vi "HouseBlend.vi"(8 "error in (no error)":errorcluster caption="错误输入（无错误）", 11 "House Blend Coffee 输入":refnum<class "House Blend Coffee.lvclass">) -> (0 "error out":errorcluster caption="错误输出", 3 "House Blend Coffee 输出":refnum<class "House Blend Coffee.lvclass">)   [LabVIEW 2016, in "House Blend Coffee.lvclass"]
uses:
  House Blend Coffee.lvclass
  Beverage.lvclass/Beverage.ctl
  Beverage.lvclass
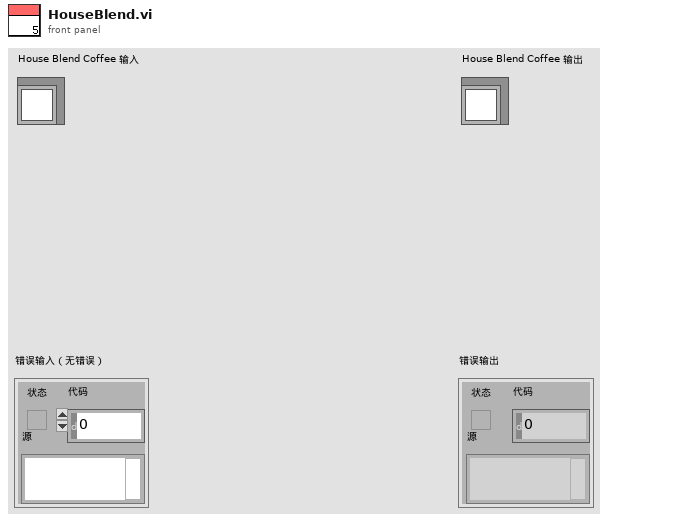
[diagram p1: front panel]
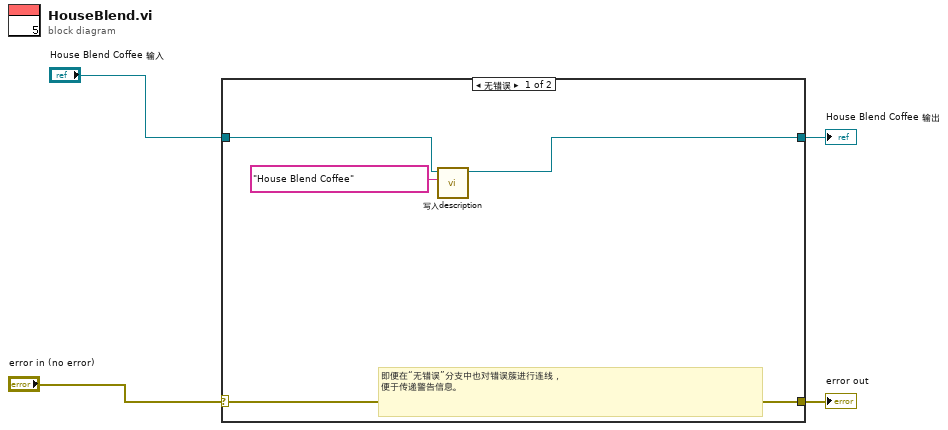
[diagram p0: block diagram]
diagram:
  n1 = case shown="无错误" "error in (no error)" {
    selector: "error in (no error)" -> [w8 w10]
    tunnel: [w8 w10] -> w3
    tunnel: [w6 w9] -> w1
    tunnel: "House Blend Coffee 输入" -> [w7 w9]
    frame No Error {
      # "即便在“无错误”分支中也对错误簇进行连线，\n便于传递警告信息。"
      n2 = call "写入description.vi"("description"="House Blend Coffee", "Beverage输入"=w7) -> ("Beverage输出"=w6:refnum<class "House Blend Coffee.lvclass">)  [unwired: 8 in, 1 out]
    }
    frame Error {
    }
  }
  "error out" <- w3
  "House Blend Coffee 输出" <- w1
